vi "ParsePacket.vi"(0 "data out":string) -> (1 "Counter":i16, 2 "Dummy":i16, 3 "Bytes read":i32)   [LabVIEW 2010]
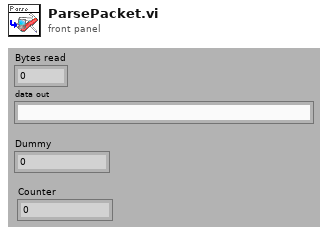
[diagram p1: front panel]
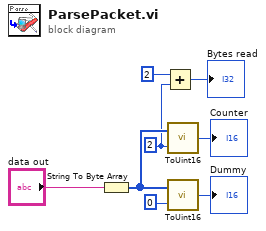
[diagram p0: block diagram]
diagram:
  w1 = 2 ("index")
  n1 = String To Byte Array(string="data out") -> (unsigned byte array=w3:u8[])
  n2 = Add(x=2, y=w1) -> (x+y=→"Bytes read":i32)
  n3 = call "ToUint16.vi"("index"=w1, "array"=w3) -> ("sp float"=→"Counter":u16)
  n4 = call "ToUint16.vi"("index"=0, "array"=w3) -> ("sp float"=→"Dummy":u16)
